vi "niRFUtil FTW Brickwall Filter (real wfm).vi"(0 "Waveform In (V)":T3 {"y" min=0 max=127 format="%.2f"; "dx" format="%^.2e"; "x0" format="%^.2e"}, 5 "Center Frequency (Hz)":dbl format="%^.6e", 7 "Bandwidth (Hz)":dbl=1000000.0 format="%^.6e") -> (4 "Waveform Out (V)":T1 {"y" format="%.2f"; "dx" format="%^.2e"; "x0" format="%^.2e"})   [LabVIEW 2015, in "niRFUtil.lvlib"]
doc: "(c) Copyright 2006, National Instruments, Inc. This VI may not be duplicated, sold, or distributed without written consent from National Instruments."
uses:
  niRFUtil.lvlib
  Includes/niRFUtil INC Real Waveform.ctl
  Includes/niRFUtil INC Real Array.ctl
  Includes/niRFUtil INC Complex Waveform.ctl
  Includes/niRFUtil INC Complex Array.ctl
  niRFUtil FTW IFFT (complex wfm).vi
  Waveform Manipulation/niRFUtil WFM Multiply Waveforms (complex wfm).vi
  Measurements/niRFUtil MEAS Waveform Statistics (complex wfm).vi
  niRFUtil FTW FFT (real wfm).vi
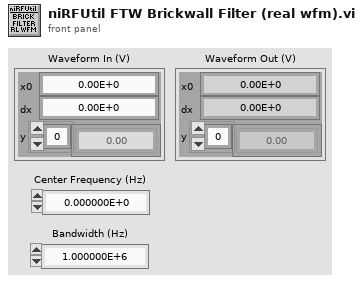
[diagram p1: front panel]
types:
  T1 = typedef "niRFUtil.lvlib/niRFUtil INC Complex Waveform.ctl" = cluster{"x0":dbl, "dx":dbl, "y":T2}
  T2 = typedef "niRFUtil.lvlib/niRFUtil INC Complex Array.ctl" = csg[]
  T3 = typedef "niRFUtil.lvlib/niRFUtil INC Real Waveform.ctl" = cluster{"x0":dbl, "dx":dbl, "y":T4}
  T4 = typedef "niRFUtil.lvlib/niRFUtil INC Real Array.ctl" = sgl[]
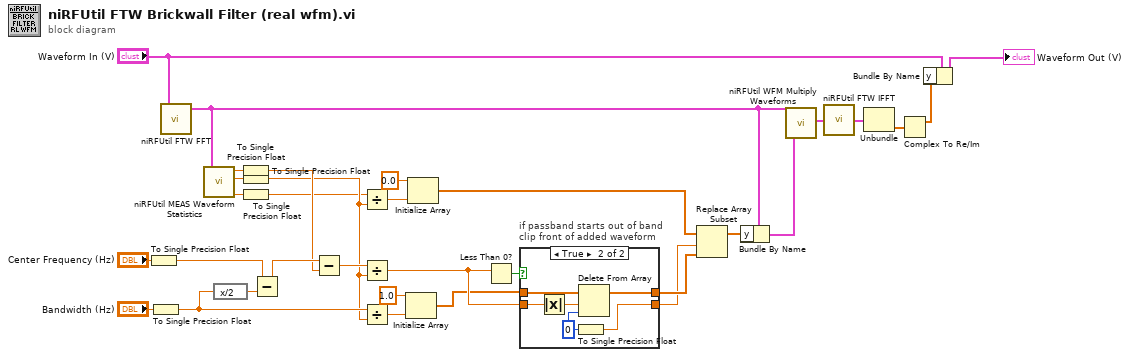
[diagram p0: block diagram]
diagram:
  n1 = To Single Precision Float(number="Center Frequency (Hz)") -> (single precision float=w6:sgl)
  n2 = To Single Precision Float(number="Bandwidth (Hz)") -> (single precision float=w5:sgl)
  n3 = call-poly "niRFUtil FTW FFT.vi"("Waveform In (V)"="Waveform In (V)") -> ("Waveform Out (V)"=w18:T1)  [unwired: 2 in, 2 out]
  n4 = call-poly "niRFUtil MEAS Waveform Statistics.vi"("Waveform In"=w18) -> ("Start"=w29:dbl, "Interval"=w22:dbl, "Duration"=w32:dbl)  [unwired: 5 out]
  n5 = expression code="x/2"(w5) -> (w25:sgl)
  n6 = To Single Precision Float(number=w29) -> (single precision float=w4:sgl)
  n7 = To Single Precision Float(number=w22) -> (single precision float=w3:sgl)
  n8 = To Single Precision Float(number=w32) -> (single precision float=w2:sgl)
  n9 = Subtract(x=w6, y=w25) -> (x-y=w24:sgl)
  n10 = Subtract(x=w24, y=w4) -> (x-y=w28:sgl)
  n11 = Divide(x=w2, y=w3) -> (x/y=w31:sgl)
  n12 = Divide(x=w28, y=w3) -> (x/y=w10:sgl)
  n13 = Divide(x=w5, y=w3) -> (x/y=w20:sgl)
  n14 = Initialize Array(sgl 1.0 ("element"), w20) -> (w9:sgl[])
  n15 = Initialize Array(sgl 0.0 ("element"), w31) -> (w27:sgl[])
  n16 = Less Than 0?(x=w10) -> (x < 0?=w12:bool)
  n17 = case "if passband starts out of band\nclip front of added waveform" shown="True" w12 {
    tunnel: w9 -> [w34 w36]
    tunnel: [w34 w40] -> w11
    tunnel: w10 -> [w33 w37]
    tunnel: [w33 w35] -> w8
    frame False {
    }
    frame True {
      w39 = 0 ("index")
      n18 = Absolute Value(x=w37) -> (abs(x)=w38:sgl)
      n19 = To Single Precision Float(number=w39) -> (single precision float=w35:sgl)
      n20 = Delete From Array(array=w36, length=w38, index=w39) -> (array with subset deleted=w40:sgl[])  [unwired: 1 out]
    }
  }
  n21 = Replace Array Subset(array=w27, new element=w11, index=w8) -> (w19:sgl[])
  n22 = Bundle By Name(cluster=w18, "y"=w19) -> (w17:T1)
  n23 = call-poly "niRFUtil WFM Multiply Waveforms.vi"("Waveform 2 In"=w17, "Waveform 1 In"=w18) -> ("Waveform Out"=w16:T1)  [unwired: 1 out]
  n24 = call-poly "niRFUtil FTW IFFT.vi"("Waveform In (V)"=w16) -> ("Waveform Out (V)"=w15:T1)
  n25 = Unbundle(w15) -> ("y"=w14:T2)  [unwired: 2 out]
  n26 = Complex To Re/Im(x + iy=w14) -> (x=w13:sgl[])  [unwired: 1 out]
  n27 = Bundle By Name(cluster="Waveform In (V)", "y"=w13) -> (→"Waveform Out (V)":T3)
